vi "Create Base Measurement Annotations.vi"(8 "error in":errorcluster, 9 "Tags":string[](array[string]), 10 "Collection":string, 11 "Description":string) -> (0 "error out":errorcluster, 3 "Measurement Annotations":T1[](array[typedef]))   [LabVIEW 2020, in "MeasurementLink Measurement Server.lvlib"]
uses:
  MeasurementLink Measurement Server.lvlib
  TypeDefs/MeasurementAnnotation.ctl
  a9ad9b04-f222-4ebf-94b5-602fd11bc15e.vi
  0221d297-ed52-46f4-bb7b-f2207ffca4d2.vi
  725c875f-b543-4029-b405-f80e7b23a3ec.vi
  a9ad9b04-f222-4ebf-94b5-602fd11bc15e.vi/77476d48-7c31-46ad-92c1-ee98bcbcef06.vi
  0221d297-ed52-46f4-bb7b-f2207ffca4d2.vi/77476d48-7c31-46ad-92c1-ee98bcbcef06.vi
  725c875f-b543-4029-b405-f80e7b23a3ec.vi/77476d48-7c31-46ad-92c1-ee98bcbcef06.vi
  <vilib>/Utility/Data Type/Get Type Information.vi
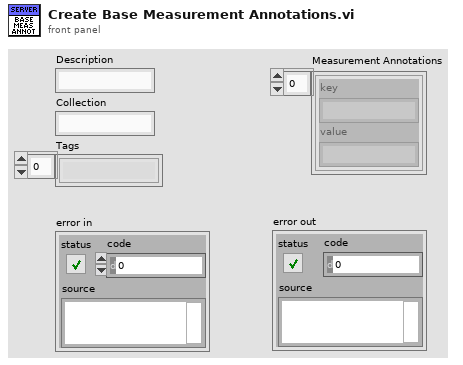
[diagram p1: front panel]
types:
  T1 = typedef "MeasurementLink Measurement Server.lvlib/MeasurementAnnotation.ctl" = cluster{"key":string, "value":string}
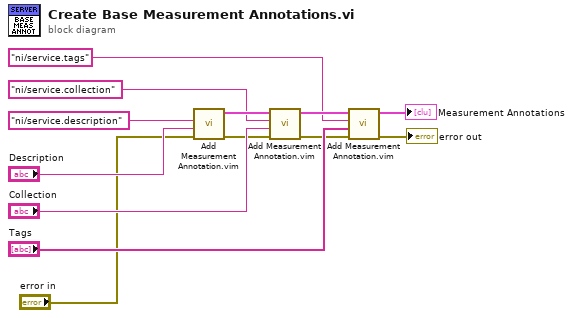
[diagram p0: block diagram]
diagram:
  n1 = call "Add Measurement Annotation.vim"("error in"="error in", "Value (anything)"="Description", "Key"="ni/service.description") -> ("error out"=w3:errorcluster, "Measurement Annotations Out"=w12:T1[])  [unwired: 7 in]
  n2 = call "Add Measurement Annotation.vim"("error in"=w3, "Value (anything)"="Collection", "Key"="ni/service.collection", "Measurement Annotations In"=w12) -> ("error out"=w4:errorcluster, "Measurement Annotations Out"=w13:T1[])  [unwired: 6 in]
  n3 = call "Add Measurement Annotation.vim"("error in"=w4, "Value (anything)"="Tags", "Key"="ni/service.tags", "Measurement Annotations In"=w13) -> ("error out"=→"error out":errorcluster, "Measurement Annotations Out"=→"Measurement Annotations":T1[])  [unwired: 6 in]
